vi "短日期时间转长日期格式.vi"(10 "table输入":string(combo), 11 "data":string[][](table)) -> (3 "输出数组":string[][](array[string]))   [LabVIEW 2016, in "数据传输系统.lvlib"]
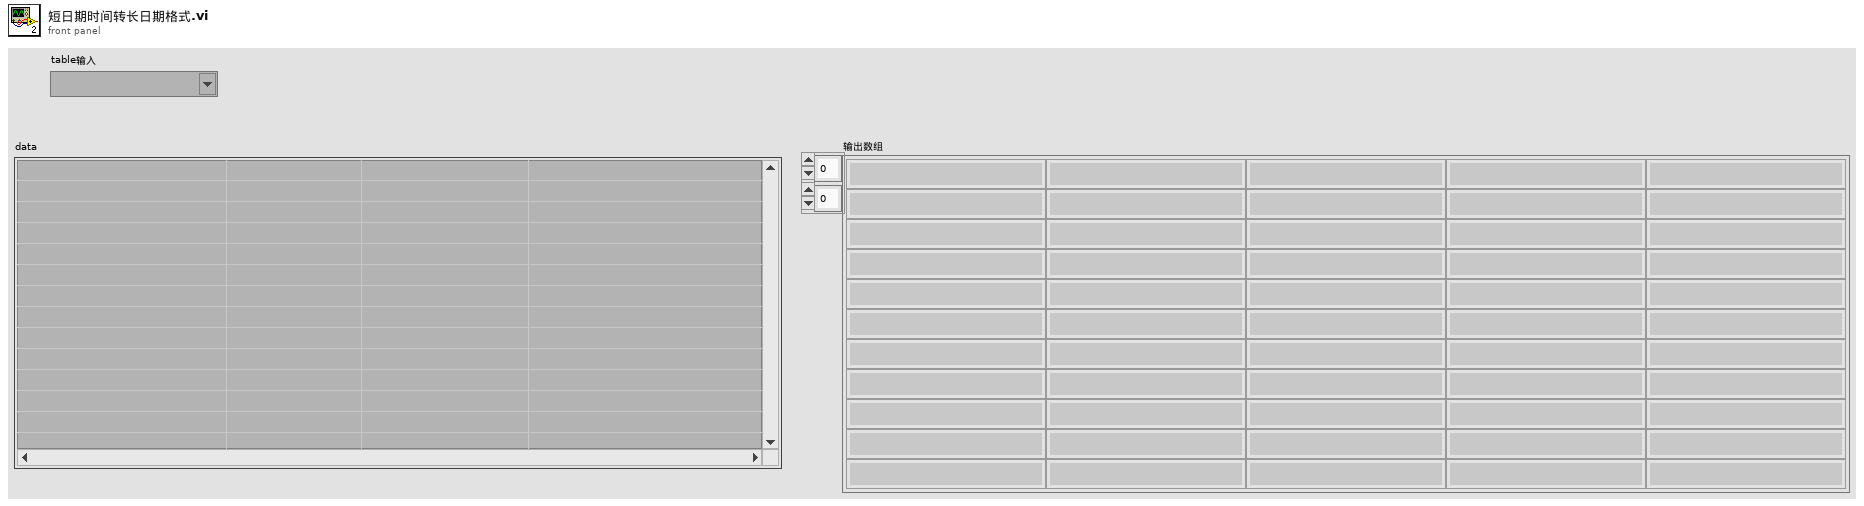
[diagram p1: front panel]
types:
  T1 = typedef "LVDateTimeRec.ctl" = cluster{"秒数的小数部分":dbl, "秒":i32, "分":i32, "时":i32, "日":i32, "月":i32, "年":i32, "天数（周）":i32, "天数（年）":i32, "DST":i32}
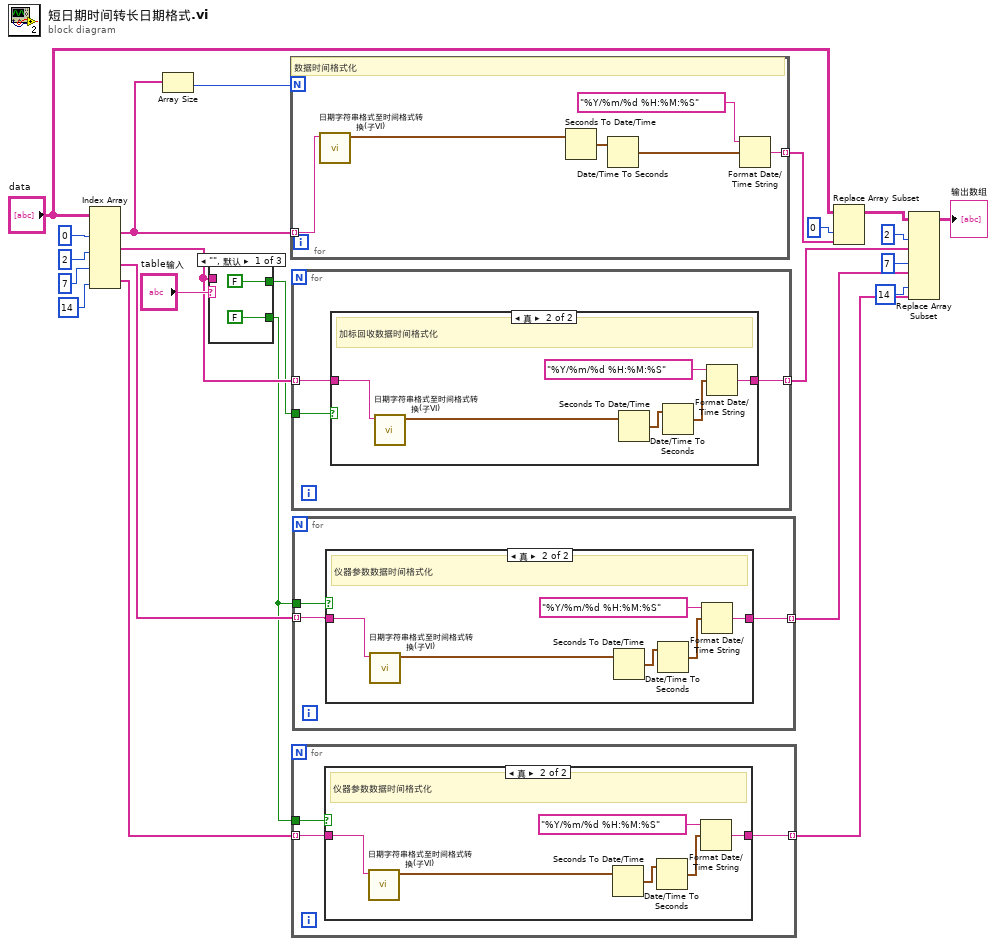
[diagram p0: block diagram]
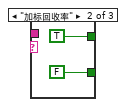
[diagram p5: hidden frame]
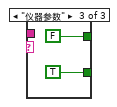
[diagram p6: hidden frame]
diagram:
  n1 = Index Array(array="data", index (col) #1=0 ("禁用的索引 (列)"), index (col) #2=2 ("索引 (列)"), index (col) #3=7 ("索引 (列)"), index (col) #4=14 ("索引 (列)")) -> (element #1=w10:string[], element #2=w8:string[], element #3=w4:string[], element #4=w5:string[])  [unwired: 4 in]
  n2 = Array Size(array=w10) -> (size(s)=w9:i32)
  n3 = case shown="\"\", 默认" "table输入" {
    tunnel: [FALSE TRUE FALSE] -> w7
    tunnel: w8 -> [_ _ _]
    tunnel: [FALSE FALSE TRUE] -> w1
    frame "", Default {
    }
    frame "加标回收率" {
    }
    frame "仪器参数" {
    }
  }
  n4 = for {
    N: w9 -> [_]
    tunnel: [w31] -> w19 mode=indexing
    tunnel: w10 -> [w30] mode=indexing
    # "数据时间格式化"
    n5 = call "日期字符串格式至时间格式转换(子VI).vi"("data[0]"=w30) -> ("time stamp"=w34:timestamp)  [unwired: 10 in]
    n6 = Seconds To Date/Time(time stamp (now)=w34) -> (date time rec=w35:T1)  [unwired: 1 in]
    n7 = Date/Time To Seconds(2:w35) -> (0:w33:timestamp)  [unwired: 1 in]
    n8 = Format Date/Time String(time format string (%c)="%Y/%m/%d %H:%M:%S" ("时间格式字符串(%c)"), seconds (now)=w33) -> (date/time string=w31:string)  [unwired: 1 in]
  }
  n9 = for {
    tunnel: w8 -> [w38] mode=indexing
    tunnel: w7 -> [w37]
    tunnel: [w36] -> w6 mode=indexing
    n10 = case shown="真" w37 {
      tunnel: [w39 w41] -> w36
      tunnel: w38 -> [w39 w40]
      frame False {
      }
      frame True {
        # "加标回收数据时间格式化"
        n11 = call "日期字符串格式至时间格式转换(子VI).vi"("data[0]"=w40) -> ("time stamp"=w43:timestamp)  [unwired: 10 in]
        n12 = Seconds To Date/Time(time stamp (now)=w43) -> (date time rec=w42:T1)  [unwired: 1 in]
        n13 = Date/Time To Seconds(2:w42) -> (0:w44:timestamp)  [unwired: 1 in]
        n14 = Format Date/Time String(time format string (%c)="%Y/%m/%d %H:%M:%S" ("时间格式字符串(%c)"), seconds (now)=w44) -> (date/time string=w41:string)  [unwired: 1 in]
      }
    }
  }
  n15 = for {
    tunnel: w5 -> [w48] mode=indexing
    tunnel: w1 -> [w47]
    tunnel: [w46] -> w3 mode=indexing
    n16 = case shown="真" w47 {
      tunnel: [w49 w51] -> w46
      tunnel: w48 -> [w49 w50]
      frame False {
      }
      frame True {
        # "仪器参数数据时间格式化"
        n17 = call "日期字符串格式至时间格式转换(子VI).vi"("data[0]"=w50) -> ("time stamp"=w53:timestamp)  [unwired: 10 in]
        n18 = Seconds To Date/Time(time stamp (now)=w53) -> (date time rec=w52:T1)  [unwired: 1 in]
        n19 = Date/Time To Seconds(2:w52) -> (0:w54:timestamp)  [unwired: 1 in]
        n20 = Format Date/Time String(time format string (%c)="%Y/%m/%d %H:%M:%S" ("时间格式字符串(%c)"), seconds (now)=w54) -> (date/time string=w51:string)  [unwired: 1 in]
      }
    }
  }
  n21 = for {
    tunnel: w4 -> [w58] mode=indexing
    tunnel: [w57] -> w2 mode=indexing
    tunnel: w1 -> [w56]
    n22 = case shown="真" w56 {
      tunnel: [w59 w61] -> w57
      tunnel: w58 -> [w59 w60]
      frame False {
      }
      frame True {
        # "仪器参数数据时间格式化"
        n23 = call "日期字符串格式至时间格式转换(子VI).vi"("data[0]"=w60) -> ("time stamp"=w63:timestamp)  [unwired: 10 in]
        n24 = Seconds To Date/Time(time stamp (now)=w63) -> (date time rec=w62:T1)  [unwired: 1 in]
        n25 = Date/Time To Seconds(2:w62) -> (0:w64:timestamp)  [unwired: 1 in]
        n26 = Format Date/Time String(time format string (%c)="%Y/%m/%d %H:%M:%S" ("时间格式字符串(%c)"), seconds (now)=w64) -> (date/time string=w61:string)  [unwired: 1 in]
      }
    }
  }
  n27 = Replace Array Subset(array="data", new element=w19, index (col)=0 ("禁用的索引 (列)")) -> (w16:string[][])  [unwired: 1 in]
  n28 = Replace Array Subset(array=w16, new element #1=w6, index (col) #1=2 ("索引 (列)"), new element #2=w2, index (col) #2=7 ("索引 (列)"), new element #3=w3, index (col) #3=14 ("索引 (列)")) -> (→"输出数组":string[][])  [unwired: 3 in]
